vi "Robot_enabled.vi"(8 "Include test mode? (F)":bool, 11 "Robot Mode in":T1) -> (3 "Enabled?":bool)   [LabVIEW 2017, in "labview-standard-library.lvlib" / "data-logging.lvlib"]
uses:
  <vilib>/Rock Robotics/WPI/DriverStation/WPI_DriverStationRobotMode2.ctl
  data-logging.lvlib
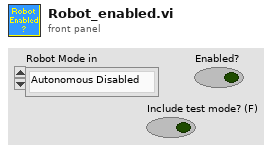
[diagram p1: front panel]
types:
  T1 = typedef "WPI_DriverStationRobotMode2.ctl" = enum16{"Autonomous Disabled", "Autonomous Enabled", "Teleop Disabled", "Teleop Enabled", "Disconnected", "Finish", "Test Disabled", "Test Enabled", "Emergency Stopped"}
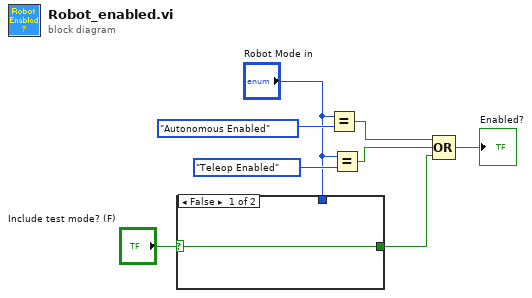
[diagram p0: block diagram]
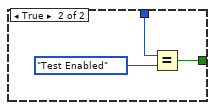
[diagram p2: hidden frame]
diagram:
  n1 = case shown="False" "Include test mode? (F)" {
    selector: "Include test mode? (F)" -> [w9 _]
    tunnel: "Robot Mode in" -> [_ w12]
    tunnel: [w9 w10] -> w2
    frame False {
    }
    frame True {
      n2 = Equal?(x=w12, y=WPI_DriverStationRobotMode2."Test Enabled" ("Robot Mode")) -> (x = y?=w10:bool)
    }
  }
  n3 = Equal?(x="Robot Mode in", y=WPI_DriverStationRobotMode2."Autonomous Enabled" ("Robot Mode")) -> (x = y?=w6:bool)
  n4 = Equal?(x="Robot Mode in", y=WPI_DriverStationRobotMode2."Teleop Enabled" ("Robot Mode")) -> (x = y?=w7:bool)
  n5 = Compound Arithmetic op=OR(w6, w7, w2) -> (→"Enabled?":bool)
